vi "ShooterControl.vi"(5 "MotorConfig":T3={"CAN Address"=0, "Invert"=FALSE, "InvertSensor"=FALSE, "Unit Conversion Factor"=0.0, "Brake Mode"=enum."Override to Brake", "Reverse Limt Switch Mode"=enum."Disabled", "Forward Limt Swith Mode"=enum."Disabled", "PWM Channel"=enum."Invalid", "Motor Controller Type"=enum."Talon SRX", "Peak Current (A)"=0, "Continuous Current (A)"=0, "Peak Duration (ms)"=0, "Current Limit Enable"=FALSE}, 6 "PIDParams":T13, 7 "Setpoint (rpm)":dbl, 8 "FollowerMotorControlDevRef":T9, 9 "LeaderMotorControlDevRef":T9) -> (2 "ShooterReady":bool, 3 "Sensor Velocity":dbl)   [LabVIEW 2019]
uses:
  <vilib>/Rock Robotics/WPI/MotorControl/WPI_MotorControlDeviceRef.ctl
  <vilib>/Rock Robotics/WPI/MotorControl/WPI_MotorControlType.ctl
  <vilib>/Rock Robotics/SystemInterfaces/DIO/FPGA_DIOPWMChannel.ctl
  <vilib>/Rock Robotics/WPI/PWM/WPI_PWMDeadband.ctl
  <vilib>/Rock Robotics/SystemInterfaces/DIO/FPGA_DIOChannel.ctl
  ArgosLib/Config/ConfigComponents/TypeDefs/Config_PIDParams.ctl
  <vilib>/Rock Robotics/WPI/ThirdParty/Phoenix-LabVIEW/Motor Controller/Controls/CTRE_Phoenix_MotorControl_ControlMode.ctl
  ArgosLib/Config/ConfigComponents/TypeDefs/Config_Motor.ctl
  <vilib>/Rock Robotics/WPI/ThirdParty/Phoenix-LabVIEW/Motor Controller/Controls/CTRE_Phoenix_MotorControl_NeutralMode.ctl
  <vilib>/Rock Robotics/WPI/ThirdParty/Phoenix-LabVIEW/Motor Controller/Controls/CTRE_Phoenix_MotorControl_LimitSwitchNormal.ctl
  ArgosLib/Config/ConfigComponents/TypeDefs/Config_MotorCtrlType.ctl
  <vilib>/Rock Robotics/WPI/ThirdParty/Phoenix-LabVIEW/Motor Controller/Controls/CTRE_Phoenix_MotorControl_Faults.ctl
  <vilib>/Rock Robotics/WPI/ThirdParty/Phoenix-LabVIEW/Motor Controller/Controls/CTRE_Phoenix_MotorControl_StickyFaults.ctl
  <vilib>/Rock Robotics/WPI/ThirdParty/Phoenix-LabVIEW/Motor Controller/Get/CTRE_Phoenix_MotorController_GetSupplyAndStatorCurrent_Enhanced.vi
  <vilib>/Rock Robotics/WPI/ThirdParty/Phoenix-LabVIEW/Motor Controller/Get/CTRE_Phoenix_MotorController_GetVoltage.vi
  <vilib>/Rock Robotics/WPI/ThirdParty/Phoenix-LabVIEW/Motor Controller/Get/CTRE_Phoenix_MotorController_GetSelectedSensorData.vi
  ArgosLib/ArgosLib.lvlib
panel:
  in  "SetpointReachedDebounce (ms)":u32=100
  in  "AllowableError (rpm)":dbl=200.0
  in  "ManualSetpoint":dbl
  in  "ManualSetpointEnable":bool
  out "FollowerStickyFaults":T1
  out "FollowerFaults":T2
  out "LeaderStickyFaults":T1
  out "LeaderFaults":T2
  in  "Control Mode":T8=2 items=["PercentOutput"=0, "Position"=1, "Velocity"=2, "Current"=3, "Follower"=5, "MotionProfile"=6, "MotionMagic"=7, "MotionProfileArc"=10, "Disabled"=15]
  out "FollowerCurrent":dbl
  out "LeaderCurrent":dbl
  in  "Use Manual PID?":bool
  in  "Manual PIDParams":T13={"P"=1.0, "I"=0.0, "D"=0.0, "F"=0.05, "IZone"=0.0}
  out "Applied Output":dbl
  out "Waveform Chart":cluster{"Sensor Velocity":dbl, "Setpoint":dbl}(graph)
  out "Sensor Position":dbl
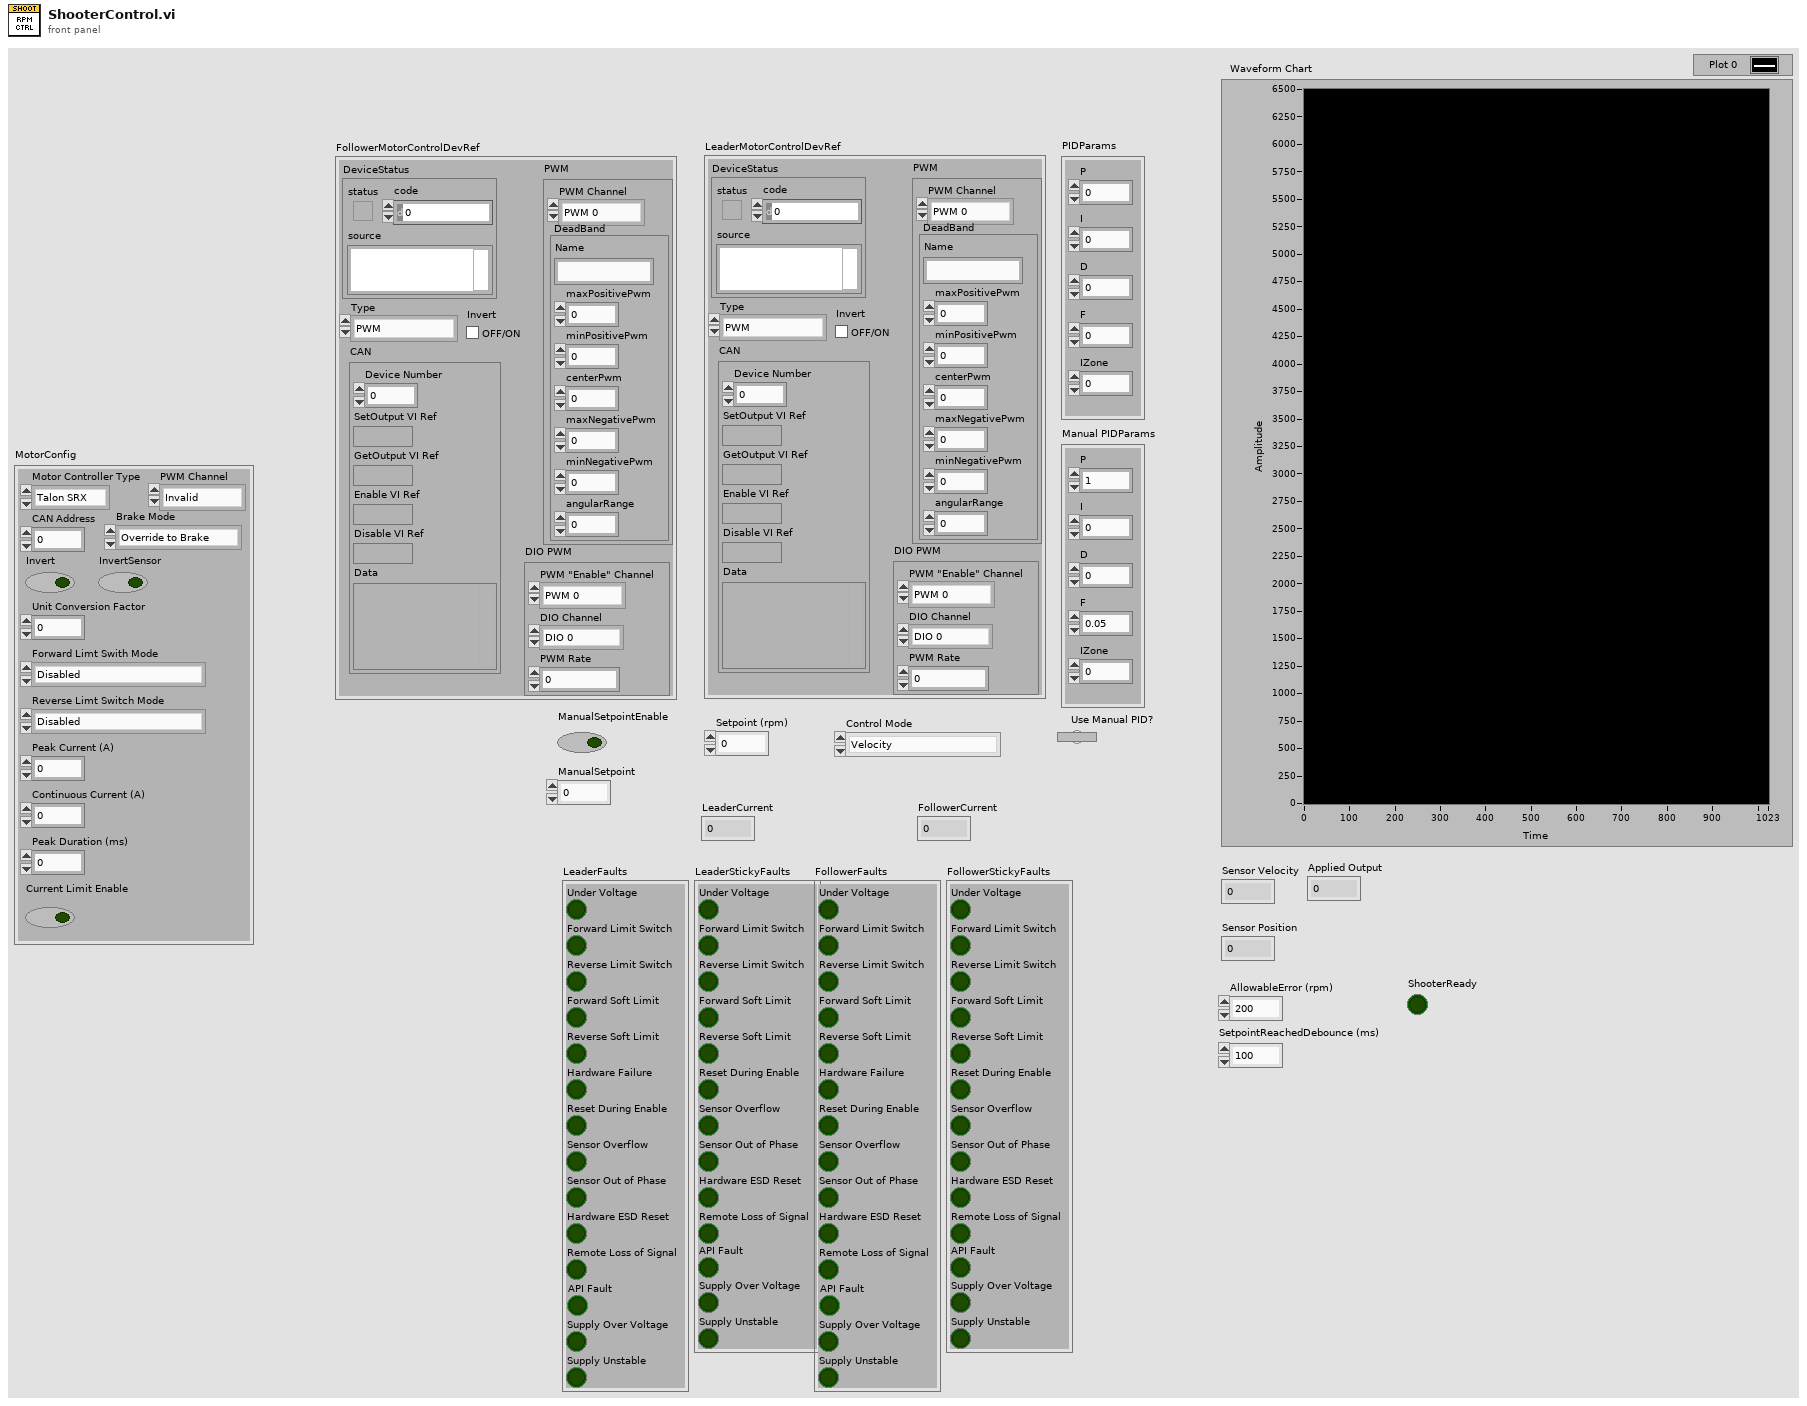
[diagram p1: front panel]
types:
  T1 = typedef "CTRE_Phoenix_MotorControl_StickyFaults.ctl" = cluster{"Under Voltage":bool, "Forward Limit Switch":bool, "Reverse Limit Switch":bool, "Forward Soft Limit":bool, "Reverse Soft Limit":bool, "Reset During Enable":bool, "Sensor Overflow":bool, "Sensor Out of Phase":bool, "Hardware ESD Reset":bool, "Remote Loss of Signal":bool, "API Fault":bool, "Supply Over Voltage":bool, "Supply Unstable":bool}
  T2 = typedef "CTRE_Phoenix_MotorControl_Faults.ctl" = cluster{"Under Voltage":bool, "Forward Limit Switch":bool, "Reverse Limit Switch":bool, "Forward Soft Limit":bool, "Reverse Soft Limit":bool, "Hardware Failure":bool, "Reset During Enable":bool, "Sensor Overflow":bool, "Sensor Out of Phase":bool, "Hardware ESD Reset":bool, "Remote Loss of Signal":bool, "API Fault":bool, "Supply Over Voltage":bool, "Supply Unstable":bool}
  T3 = typedef "ArgosLib.lvlib/Config_Motor.ctl" = cluster{"CAN Address":u8, "Invert":bool, "InvertSensor":bool, "Unit Conversion Factor":dbl, "Brake Mode":T4, "Reverse Limt Switch Mode":T5, "Forward Limt Swith Mode":T5, "PWM Channel":T6, "Motor Controller Type":T7, "Peak Current (A)":i32, "Continuous Current (A)":i32, "Peak Duration (ms)":i32, "Current Limit Enable":bool}
  T4 = typedef "CTRE_Phoenix_MotorControl_NeutralMode.ctl" = enum8{"EEPROMSetting", "Override to Coast", "Override to Brake"}
  T5 = typedef "CTRE_Phoenix_MotorControl_LimitSwitchNormal.ctl" = enum16{"Normally Open", "Normally Closed", "Disabled"}
  T6 = typedef "FPGA_DIOPWMChannel.ctl" = enum8{"PWM 0", "PWM 1", "PWM 2", "PWM 3", "PWM 4", "PWM 5", "PWM 6", "PWM 7", "PWM 8", "PWM 9", "PWM MXP 0", "PWM MXP 1", "PWM MXP 2", "PWM MXP 3", "PWM MXP 4", "PWM MXP 5", "PWM MXP 6", "PWM MXP 7", "PWM MXP 8", "PWM MXP 9", "Invalid"}
  T7 = typedef "ArgosLib.lvlib/Config_MotorCtrlType.ctl" = enum16{"Disabled", "Talon SRX", "Talon SR", "Venom", "Spark MAX", "Falcon FX"}
  T8 = typedef "CTRE_Phoenix_MotorControl_ControlMode.ctl" = u16
  T9 = typedef "WPI_MotorControlDeviceRef.ctl" = cluster{"DeviceStatus":errorcluster, "Type":T10, "PWM":cluster{"PWM Channel":T6, "DeadBand":T11}, "CAN":cluster{"Device Number":u8, "SetOutput VI Ref":variant, "GetOutput VI Ref":variant, "Enable VI Ref":variant, "Disable VI Ref":variant, "Data":variant}, "Invert":bool, "DIO PWM":cluster{"PWM \"Enable\" Channel":T6, "DIOChannel":T12, "PWM Rate":dbl}}
  T10 = typedef "WPI_MotorControlType.ctl" = enum16{"PWM", "CAN", "DIO PWM"}
  T11 = typedef "WPI_PWMDeadband.ctl" = cluster{"Name":string, "maxPositivePwm":i32, "minPositivePwm":i32, "centerPwm":i32, "maxNegativePwm":i32, "minNegativePwm":i32, "angularRange":u16}
  T12 = typedef "FPGA_DIOChannel.ctl" = enum8{"DIO 0", "DIO 1", "DIO 2", "DIO 3", "DIO 4", "DIO 5", "DIO 6", "DIO 7", "DIO 8", "DIO 9", "DIO MXP 0", "DIO MXP 1", "DIO MXP 2", "DIO MXP 3", "DIO MXP 4", "DIO MXP 5", "DIO MXP 6", "DIO MXP 7", "DIO MXP 8", "DIO MXP 9", "DIO MXP 10", "DIO MXP 11", "DIO MXP 12", "DIO MXP 13", "DIO MXP 14", "DIO MXP 15", "SPI Port CS1", "SPI Port CS2", "SPI Port CS3", "SPI Port MISO", "SPI Port MOSI", "Invalid"}
  T13 = typedef "ArgosLib.lvlib/Config_PIDParams.ctl" = cluster{"P":dbl, "I":dbl, "D":dbl, "F":dbl, "IZone":dbl}
  T14 = cluster{"P":bool, "I":bool, "D":bool, "F":bool, "IZone":bool}
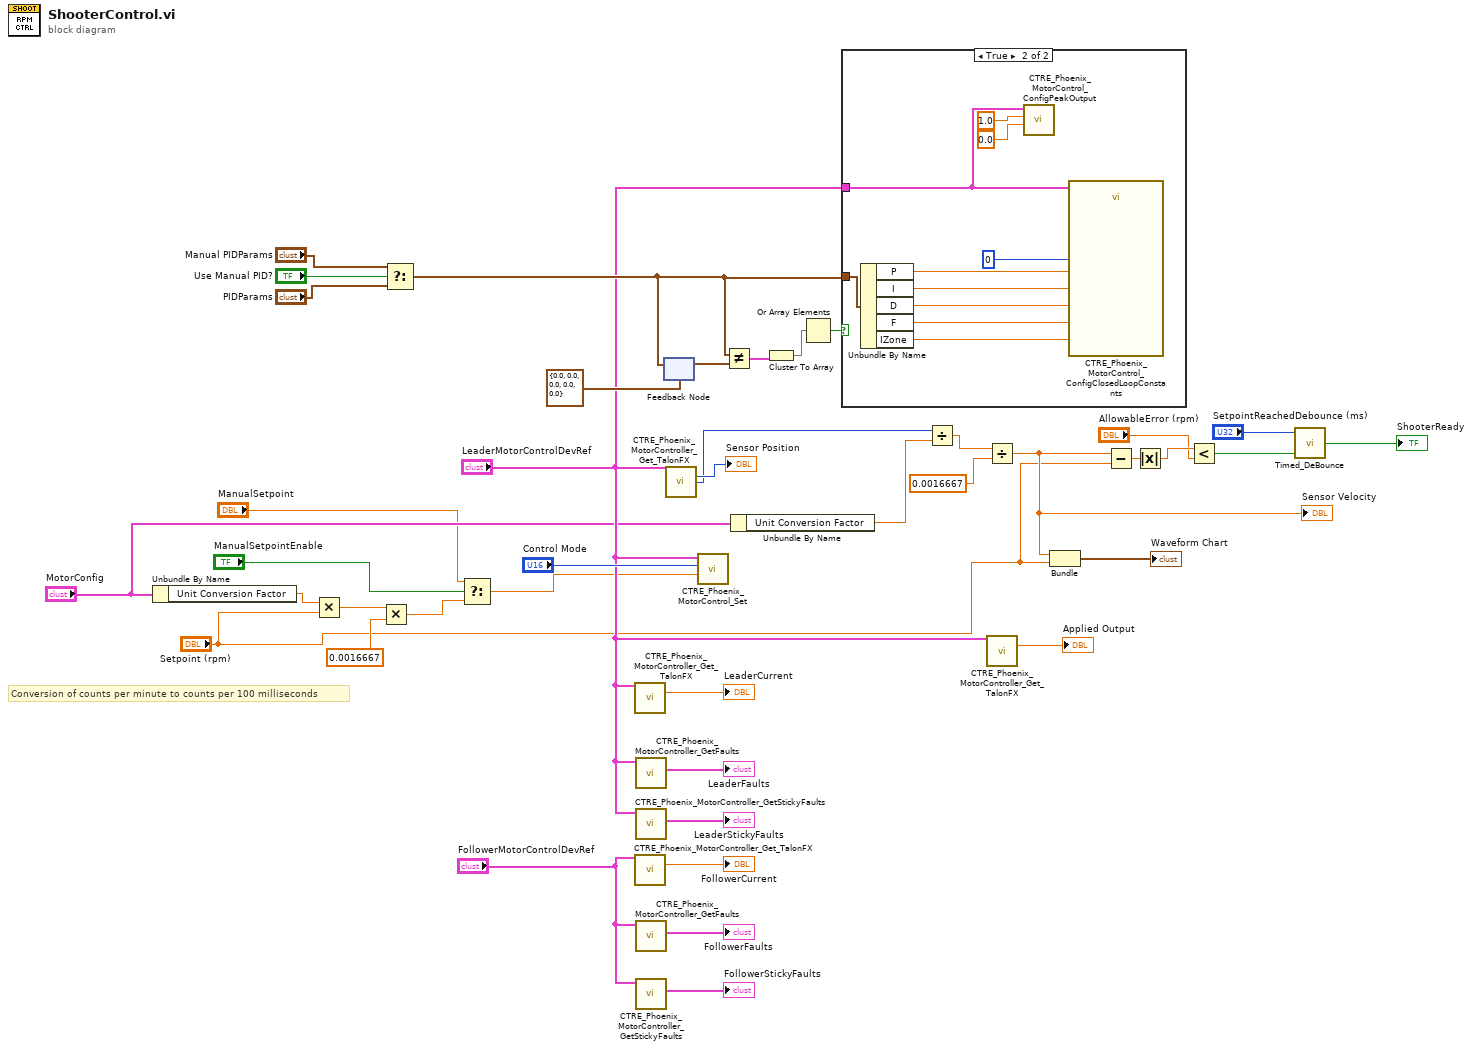
[diagram p0: block diagram]
diagram:
  # "Conversion of counts per minute to counts per 100 milliseconds"
  n1 = Unbundle By Name("MotorConfig") -> ("Unit Conversion Factor"=w31:dbl)
  n2 = Multiply(x=w31, y="Setpoint (rpm)") -> (x*y=w30:dbl)
  n3 = Multiply(x=w30, y=0.0016667) -> (x*y=w12:dbl)
  n4 = Select(t="Manual PIDParams", s="Use Manual PID?", f="PIDParams") -> (s? t:f=w34:T13)
  n5 = Select(t="ManualSetpoint", s="ManualSetpointEnable", f=w12) -> (s? t:f=w11:dbl)
  n6 = call-poly <vilib>:"CTRE_Phoenix_MotorController_Get_TalonFX.vi"("PhoenixMotorControlDevRef"="LeaderMotorControlDevRef") -> ("Supply Current"=→"LeaderCurrent":dbl)  [unwired: 11 in, 3 out]
  n7 = call-poly <vilib>:"CTRE_Phoenix_MotorController_Get_TalonFX.vi"("PhoenixMotorControlDevRef"="FollowerMotorControlDevRef") -> ("Supply Current"=→"FollowerCurrent":dbl)  [unwired: 11 in, 3 out]
  n8 = call <vilib>:"CTRE_Phoenix_MotorController_GetFaults.vi"("PhoenixMotorControlDevRef"="LeaderMotorControlDevRef") -> ("Faults"=→"LeaderFaults":T2)  [unwired: 8 in, 2 out]
  n9 = call <vilib>:"CTRE_Phoenix_MotorController_GetStickyFaults.vi"("PhoenixMotorControlDevRef"="LeaderMotorControlDevRef") -> ("Sticky Faults"=→"LeaderStickyFaults":T1)  [unwired: 8 in, 2 out]
  n10 = call <vilib>:"CTRE_Phoenix_MotorController_GetFaults.vi"("PhoenixMotorControlDevRef"="FollowerMotorControlDevRef") -> ("Faults"=→"FollowerFaults":T2)  [unwired: 8 in, 2 out]
  n11 = call <vilib>:"CTRE_Phoenix_MotorController_GetStickyFaults.vi"("PhoenixMotorControlDevRef"="FollowerMotorControlDevRef") -> ("Sticky Faults"=→"FollowerStickyFaults":T1)  [unwired: 8 in, 2 out]
  n12 = feedback #1(T13 {"P"=0.0, "I"=0.0, "D"=0.0, "F"=0.0, "IZone"=0.0} ("PIDParams")) -> (w38:T13)
  n13 = feedback-in #1(w34) -> ()
  n14 = call-poly <vilib>:"CTRE_Phoenix_MotorController_Get_TalonFX.vi"("PhoenixMotorControlDevRef"="LeaderMotorControlDevRef") -> ("Position (Raw Sensor Units)"=→"Sensor Position":i32, "Velocity (Raw Sensor Units per 100 ms)"=w27:i32)  [unwired: 11 in, 2 out]
  n15 = call <vilib>:"CTRE_Phoenix_MotorControl_Set.vi"("Output"=w11, "Control Mode"="Control Mode", "PhoenixMotorControlDevRef"="LeaderMotorControlDevRef") -> ()  [unwired: 7 in, 2 out]
  n16 = Not Equal?(x=w34, y=w38) -> (x != y?=w39:T14)
  n17 = Unbundle By Name("MotorConfig") -> ("Unit Conversion Factor"=w14:dbl)
  n18 = Cluster To Array(cluster=w39) -> (array=w41:bool[])
  n19 = Or Array Elements(Boolean array=w41) -> (logical OR=w40:bool)
  n20 = case shown="True" w40 {
    tunnel: w34 -> [_ w51]
    tunnel: "LeaderMotorControlDevRef" -> [_ w44]
    frame False {
    }
    frame True {
      n21 = Unbundle By Name(w51) -> ("P"=w50:dbl, "I"=w49:dbl, "D"=w48:dbl, "F"=w47:dbl, "IZone"=w46:dbl)
      n22 = call <vilib>:"CTRE_Phoenix_MotorControl_ConfigPeakOutput.vi"("Reverse Peak Percent Output"=0.0, "Forward Peak Percent Output"=1.0, "PhoenixMotorControlDevRef"=w44) -> ()  [unwired: 7 in, 2 out]
      n23 = call <vilib>:"CTRE_Phoenix_MotorControl_ConfigClosedLoopConstants.vi"("PhoenixMotorControlDevRef"=w44, "slotIdx"=0, "P"=w50, "I"=w49, "D"=w48, "F"=w47, "I Zone"=w46) -> ()  [unwired: 7 in, 2 out]
    }
  }
  n24 = Divide(x=w27, y=w14) -> (x/y=w26:dbl)
  n25 = Divide(x=w26, y=0.0016667) -> (x/y=w8:dbl)
  "Sensor Velocity" <- w8
  n26 = call-poly <vilib>:"CTRE_Phoenix_MotorController_Get_TalonFX.vi"("PhoenixMotorControlDevRef"="LeaderMotorControlDevRef") -> ("Percent Output"=→"Applied Output":dbl)  [unwired: 10 in, 4 out]
  n27 = Bundle(w8, "Setpoint (rpm)"="Setpoint (rpm)") -> (→"Waveform Chart":cluster{dbl, "Setpoint (rpm)":dbl})  [unwired: 1 in]
  n28 = Subtract(x=w8, y="Setpoint (rpm)") -> (x-y=w6:dbl)
  n29 = Absolute Value(x=w6) -> (abs(x)=w2:dbl)
  n30 = Less?(x=w2, y="AllowableError (rpm)") -> (x < y?=w5:bool)
  n31 = call "Timed_DeBounce.vi"("Input"=w5, "Hold Time(ms)"="SetpointReachedDebounce (ms)") -> ("Output"=→"ShooterReady":bool)  [unwired: 1 in]
